vi "Finish.vi"(8 "error in (no error)":errorcluster, 11 "Cargo Concrete in":refnum<class "Cargo Concrete.lvclass">) -> (0 "error out":errorcluster, 3 "Cargo Concrete out":refnum<class "Cargo Concrete.lvclass">)   [LabVIEW 2019, in "Cargo.lvlib" / "Cargo Concrete.lvclass"]
uses:
  Cargo Concrete.lvclass
  Cargo.lvclass
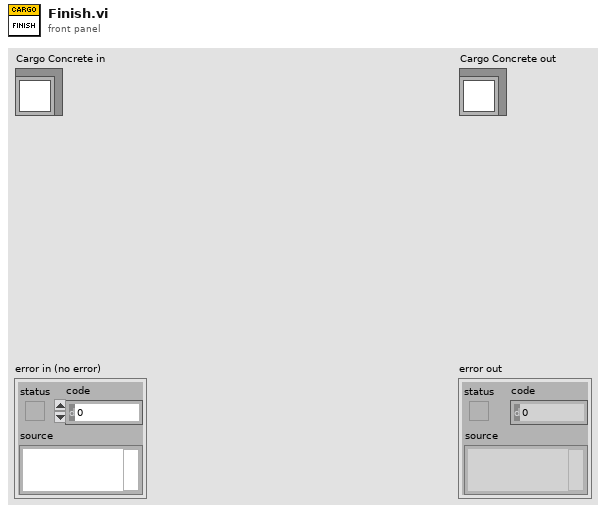
[diagram p1: front panel]
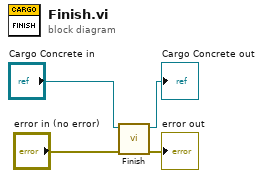
[diagram p0: block diagram]
diagram:
  n1 = call-parent "Finish.vi"("error in (no error)"="error in (no error)", "Cargo in"="Cargo Concrete in") -> ("error out"=→"error out":errorcluster, "Cargo out"=→"Cargo Concrete out":refnum<class "Cargo Concrete.lvclass">)  [unwired: 8 in]
